vi "BIN_PAQ_Concat_PAQ_samples.vi"(6 "Reversed":bool, 7 "Memory TAGs":string[](array[string]), 8 "error in (no error)":errorcluster, 9 "Added samples TAGs":string[](array[string]), 10 "PAQ Samples to ADD":T1, 11 "PAQ Samples IN":T1) -> (0 "error out":errorcluster, 3 "PAQ Samples OUT":T1)   [LabVIEW 2020, in "Sgraph_lib_V1.lvlib" / "DBAL-BIN.lvclass"]
doc: "Andre Koelewijn, 7 mar 2021\n\nThis vi will concatenate PAQ samples based on a PAQ taglist of the samples as it is required for loading in FAMM memory. This routine will add the content based on newest data first. It will subsequenctly expect data chuncks going back in time for every iteration."
uses:
  DBAL-BIN.lvclass
  controls/BIN/BINdata.ctl
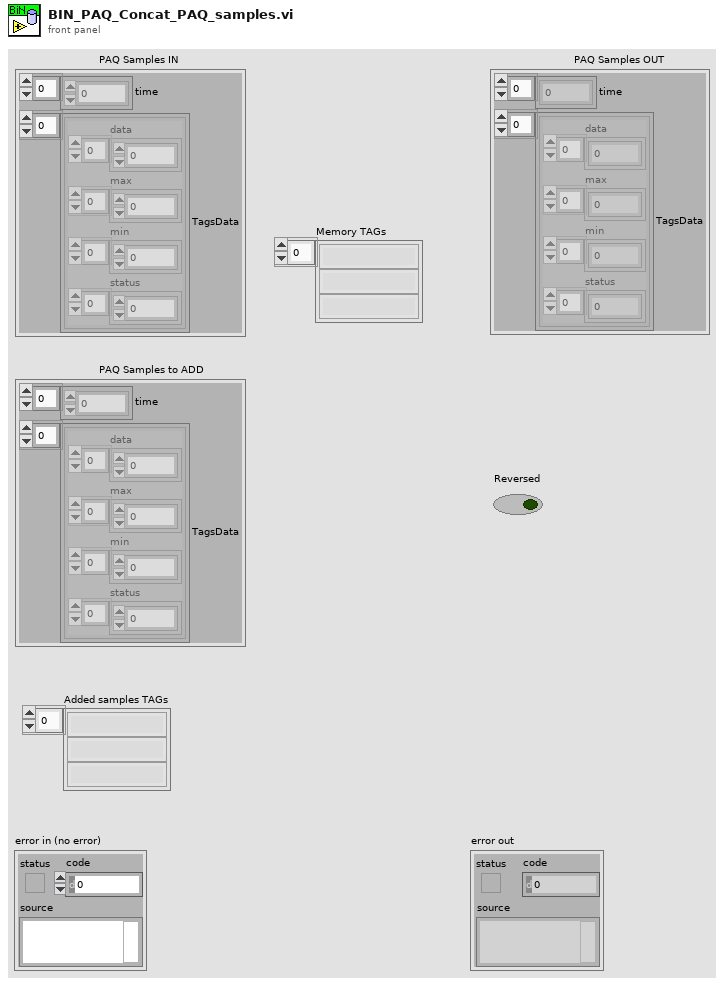
[diagram p1: front panel]
types:
  T1 = typedef "Sgraph_lib_V1.lvlib/DBAL-BIN.lvclass/BINdata.ctl" = cluster{"time":dbl[], "TagsData":cluster{"data":dbl[], "max":dbl[], "min":dbl[], "status":u32[]}[]}
  T2 = cluster{"data":dbl[], "max":dbl[], "min":dbl[], "status":u32[]}[]
  T3 = cluster{"data":dbl[], "max":dbl[], "min":dbl[], "status":u32[]}
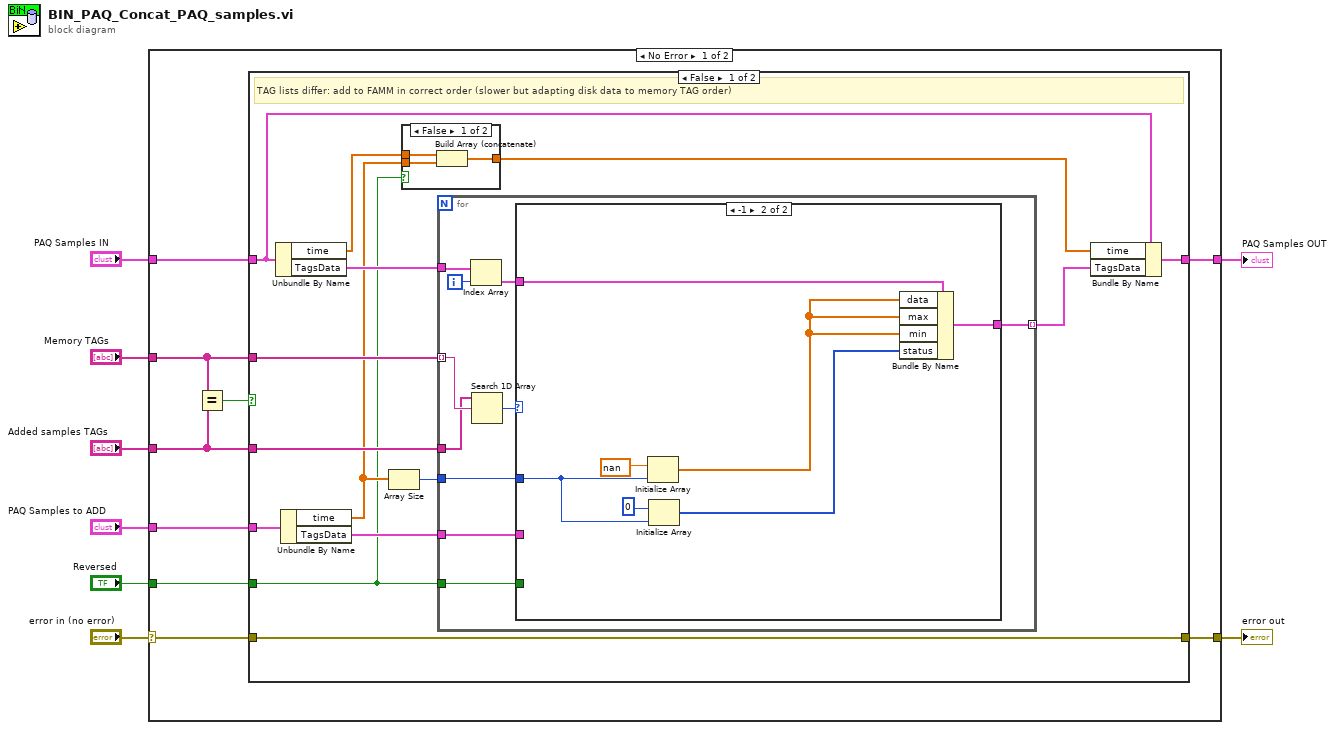
[diagram p0: block diagram]
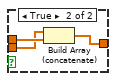
[diagram p2: hidden frame]
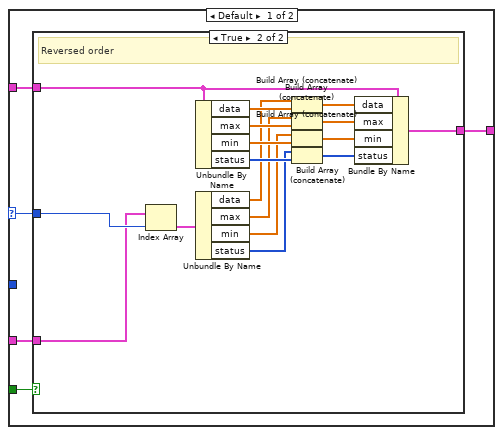
[diagram p3: hidden frame]
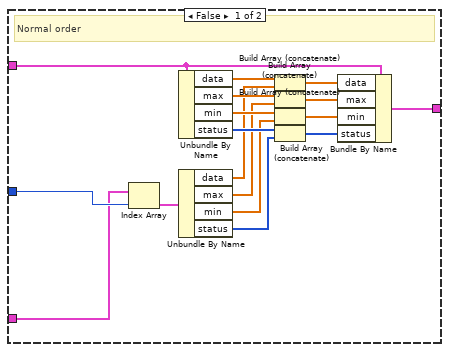
[diagram p4: hidden frame]
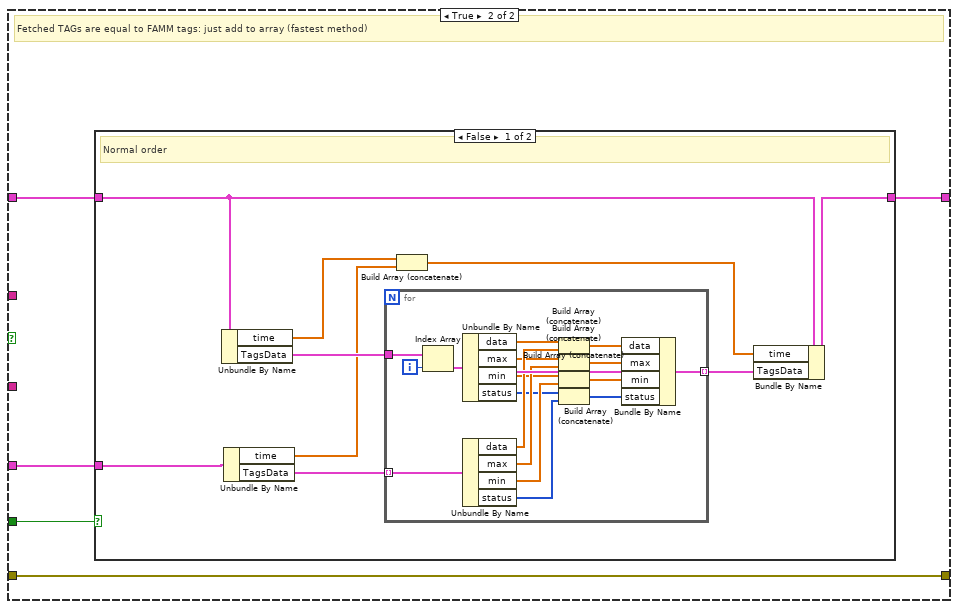
[diagram p5: hidden frame]
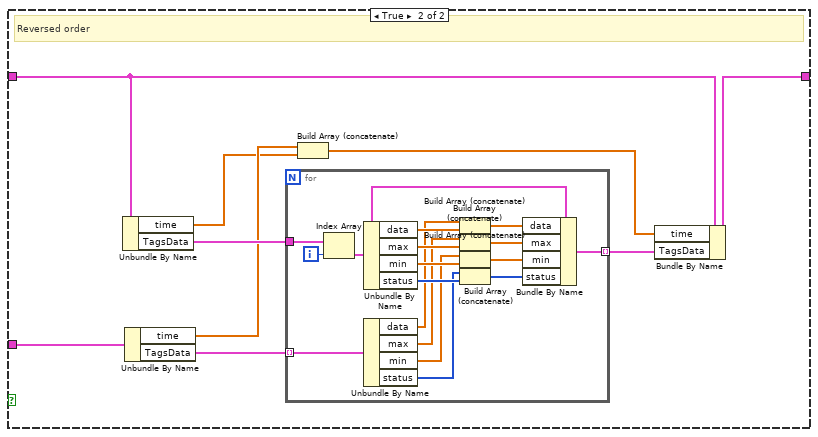
[diagram p6: hidden frame]
diagram:
  n1 = case shown="No Error" "error in (no error)" {
    selector: "error in (no error)" -> [w16 w152]
    tunnel: [w14 w152] -> w7
    tunnel: "PAQ Samples IN" -> [w17 w151]
    tunnel: [w15 w151] -> w5
    tunnel: "Memory TAGs" -> [w11 _]
    tunnel: "Added samples TAGs" -> [w12 _]
    tunnel: "PAQ Samples to ADD" -> [w13 _]
    tunnel: "Reversed" -> [w9 _]
    frame No Error {
      n2 = Equal?(x=w11, y=w12) -> (x = y?=w10:bool)
      n3 = case shown="False" w10 {
        tunnel: w17 -> [w20 w96]
        tunnel: w16 -> [w31 w98]
        tunnel: [w21 w97] -> w15
        tunnel: [w31 w98] -> w14
        tunnel: w13 -> [w27 w95]
        tunnel: w12 -> [w30 _]
        tunnel: w11 -> [w29 _]
        tunnel: w9 -> [w18 w94]
        frame False {
          # "TAG lists differ: add to FAMM in correct order (slower but adapting disk data to memory TAG order)"
          n4 = Unbundle By Name(w20) -> ("time"=w28:dbl[], "TagsData"=w25:T2)
          n5 = Unbundle By Name(w27) -> ("time"=w19:dbl[], "TagsData"=w22:T2)
          n6 = Array Size(array=w19) -> (size(s)=w23:i32)
          n7 = case shown="False" w18 {
            tunnel: w28 -> [w34 w36]
            tunnel: [w32 w37] -> w26
            tunnel: w19 -> [w33 w35]
            frame False {
              n8 = Build Array (concatenate)(w34, w33) -> (w32:dbl[])
            }
            frame True {
              n9 = Build Array (concatenate)(w35, w36) -> (w37:dbl[])
            }
          }
          n10 = for {
            tunnel: w30 -> [w42]
            tunnel: w29 -> [w46] mode=indexing
            tunnel: w25 -> [w45]
            tunnel: [w41] -> w24 mode=indexing
            tunnel: w23 -> [w40]
            tunnel: w22 -> [w39]
            tunnel: w18 -> [w38]
            i -> [w44]
            n11 = Index Array(array=w45, index=w44) -> (element=w43:T3)
            n12 = Search 1D Array(1D array=w42, element=w46) -> (index of element=w47:i32)  [unwired: 1 in]
            n13 = case shown="-1" w47 {
              selector: w47 -> [w52 _]
              tunnel: w43 -> [w50 w92]
              tunnel: [w51 w93] -> w41
              tunnel: w40 -> [_ w89]
              tunnel: w39 -> [w49 _]
              tunnel: w38 -> [w48 _]
              frame Default {
                n14 = case shown="True" w48 {
                  tunnel: w52 -> [w55 w78]
                  tunnel: [w53 w77] -> w51
                  tunnel: w50 -> [w56 w76]
                  tunnel: w49 -> [w54 w75]
                  frame False {
                    # "Normal order"
                    n15 = Index Array(array=w54, index=w55) -> (element=w61:T3)
                    n16 = Unbundle By Name(w56) -> ("data"=w62:dbl[], "max"=w63:dbl[], "min"=w64:dbl[], "status"=w65:u32[])
                    n17 = Unbundle By Name(w61) -> ("data"=w57:dbl[], "max"=w58:dbl[], "min"=w59:dbl[], "status"=w60:u32[])
                    n18 = Build Array (concatenate)(w62, w57) -> (w68:dbl[])
                    n19 = Build Array (concatenate)(w63, w58) -> (w67:dbl[])
                    n20 = Build Array (concatenate)(w64, w59) -> (w66:dbl[])
                    n21 = Build Array (concatenate)(w65, w60) -> (w69:u32[])
                    n22 = Bundle By Name(cluster=w56, "data"=w68, "max"=w67, "min"=w66, "status"=w69) -> (w53:T3)
                  }
                  frame True {
                    # "Reversed order"
                    n23 = Index Array(array=w75, index=w78) -> (element=w74:T3)
                    n24 = Unbundle By Name(w76) -> ("data"=w79:dbl[], "max"=w80:dbl[], "min"=w81:dbl[], "status"=w82:u32[])
                    n25 = Unbundle By Name(w74) -> ("data"=w73:dbl[], "max"=w72:dbl[], "min"=w71:dbl[], "status"=w70:u32[])
                    n26 = Build Array (concatenate)(w73, w79) -> (w85:dbl[])
                    n27 = Build Array (concatenate)(w72, w80) -> (w84:dbl[])
                    n28 = Build Array (concatenate)(w71, w81) -> (w83:dbl[])
                    n29 = Build Array (concatenate)(w70, w82) -> (w86:u32[])
                    n30 = Bundle By Name(cluster=w76, "data"=w85, "max"=w84, "min"=w83, "status"=w86) -> (w77:T3)
                  }
                }
              }
              frame -1 {
                n31 = Initialize Array(nan ("value"), w89) -> (w90:dbl[])
                n32 = Initialize Array(u32 0 ("value"), w89) -> (w87:u32[])
                n33 = Bundle By Name(cluster=w92, "data"=w90, "max"=w90, "min"=w90, "status"=w87) -> (w93:T3)
              }
            }
          }
          n34 = Bundle By Name(cluster=w20, "time"=w26, "TagsData"=w24) -> (w21:T1)
        }
        frame True {
          # "Fetched TAGs are equal to FAMM tags: just add to array (fastest method)"
          n35 = case shown="False" w94 {
            tunnel: [w101 w129] -> w97
            tunnel: w96 -> [w100 w128]
            tunnel: w95 -> [w99 w127]
            frame False {
              # "Normal order"
              n36 = Unbundle By Name(w100) -> ("time"=w103:dbl[], "TagsData"=w105:T2)
              n37 = Unbundle By Name(w99) -> ("time"=w102:dbl[], "TagsData"=w104:T2)
              n38 = for {
                tunnel: w104 -> [w122] mode=indexing
                tunnel: w105 -> [w124]
                tunnel: [w120] -> w106 mode=indexing
                i -> [w123]
                n39 = Index Array(array=w124, index=w123) -> (element=w121:T3)
                n40 = Unbundle By Name(w121) -> ("data"=w114:dbl[], "max"=w112:dbl[], "min"=w110:dbl[], "status"=w108:u32[])
                n41 = Unbundle By Name(w122) -> ("data"=w115:dbl[], "max"=w113:dbl[], "min"=w111:dbl[], "status"=w109:u32[])
                n42 = Build Array (concatenate)(w114, w115) -> (w117:dbl[])
                n43 = Build Array (concatenate)(w112, w113) -> (w118:dbl[])
                n44 = Build Array (concatenate)(w110, w111) -> (w119:dbl[])
                n45 = Build Array (concatenate)(w108, w109) -> (w116:u32[])
                n46 = Bundle By Name(cluster=w121, "data"=w117, "max"=w118, "min"=w119, "status"=w116) -> (w120:T3)
              }
              n47 = Build Array (concatenate)(w103, w102) -> (w107:dbl[])
              n48 = Bundle By Name(cluster=w100, "time"=w107, "TagsData"=w106) -> (w101:T1)
            }
            frame True {
              # "Reversed order"
              n49 = Unbundle By Name(w128) -> ("time"=w125:dbl[], "TagsData"=w131:T2)
              n50 = Unbundle By Name(w127) -> ("time"=w126:dbl[], "TagsData"=w130:T2)
              n51 = for {
                tunnel: w130 -> [w148] mode=indexing
                tunnel: w131 -> [w150]
                tunnel: [w146] -> w132 mode=indexing
                i -> [w149]
                n52 = Index Array(array=w150, index=w149) -> (element=w147:T3)
                n53 = Unbundle By Name(w147) -> ("data"=w141:dbl[], "max"=w140:dbl[], "min"=w139:dbl[], "status"=w138:u32[])
                n54 = Unbundle By Name(w148) -> ("data"=w137:dbl[], "max"=w136:dbl[], "min"=w135:dbl[], "status"=w134:u32[])
                n55 = Build Array (concatenate)(w137, w141) -> (w143:dbl[])
                n56 = Build Array (concatenate)(w136, w140) -> (w144:dbl[])
                n57 = Build Array (concatenate)(w135, w139) -> (w145:dbl[])
                n58 = Build Array (concatenate)(w134, w138) -> (w142:u32[])
                n59 = Bundle By Name(cluster=w147, "data"=w143, "max"=w144, "min"=w145, "status"=w142) -> (w146:T3)
              }
              n60 = Build Array (concatenate)(w126, w125) -> (w133:dbl[])
              n61 = Bundle By Name(cluster=w128, "time"=w133, "TagsData"=w132) -> (w129:T1)
            }
          }
        }
      }
    }
    frame Error {
    }
  }
  "error out" <- w7
  "PAQ Samples OUT" <- w5
